vi "Ex2.vi"   [LabVIEW 2012]
doc: "Example VI: Opens and closes Baxter's grippers"
uses:
  ROS/Code/SubVIs/BaxterSide.ctl
panel:
  # "Hit run to close and open the gripper"
types:
  T1 = typedef "BaxterSide.ctl" = enum16{"left", "right"}
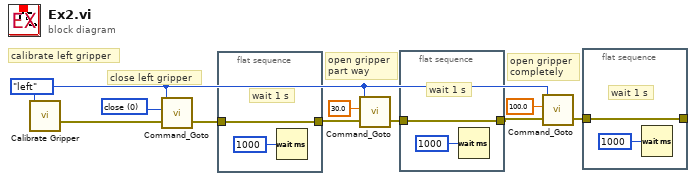
[diagram p0: block diagram]
diagram:
  w10 = u16 0 items=["close"=0, "open"=100] ("left gripper")
  w1 = BaxterSide."left" ("Side")
  # "open gripper\ncompletely"
  # "open gripper\npart way"
  # "close left gripper"
  # "calibrate left gripper"
  n1 = call "Calibrate Gripper.vi"("Side"=w1) -> ("error out"=w9:errorcluster)  [unwired: 5 in]
  n2 = call "Command_Goto.vi"("Side"=w1, "Desired Position"=w10, "error in"=w9) -> ("error out"=w7:errorcluster)  [unwired: 3 in]
  n3 = flat-sequence {
    tunnel: [w11] -> w8
    tunnel: w7 -> [w11]
    frame #0 {
      # "wait 1 s"
      n4 = Wait (ms)(milliseconds to wait=u32 1000) -> ()  [unwired: 1 out]
    }
  }
  n5 = call "Command_Goto.vi"("Side"=w1, "Desired Position"=sgl 30.0, "error in"=w8) -> ("error out"=w5:errorcluster)  [unwired: 3 in]
  n6 = flat-sequence {
    tunnel: [w13] -> w2
    tunnel: w5 -> [w13]
    frame #0 {
      # "wait 1 s"
      n7 = Wait (ms)(milliseconds to wait=u32 1000) -> ()  [unwired: 1 out]
    }
  }
  n8 = call "Command_Goto.vi"("Side"=w1, "Desired Position"=sgl 100.0, "error in"=w2) -> ("error out"=w4:errorcluster)  [unwired: 3 in]
  n9 = flat-sequence {
    tunnel: [w15] -> _
    tunnel: w4 -> [w15]
    frame #0 {
      # "wait 1 s"
      n10 = Wait (ms)(milliseconds to wait=u32 1000) -> ()  [unwired: 1 out]
    }
  }
